vi "GetGraphics.vi"(0 "LcPictureBox in":refnum<class "LcPictureBox.lvclass">, 5 "error in (no error)":errorcluster, 8 "SmoothingMode":T1) -> (14 "LcPictureBox out":refnum<class "LcPictureBox.lvclass">, 16 "Graphics":refnum<k24>, 17 "Scale":dbl, 18 "Offset":cluster{"x":sgl, "y":sgl}, 19 "error out":errorcluster)   [LabVIEW 2020, in "LcPictureBox.lvclass"]
uses:
  LcPictureBox.lvclass
  System.Drawing
  SmoothingMode.ctl
  LcPictureBox.lvclass/LcPictureBox.ctl
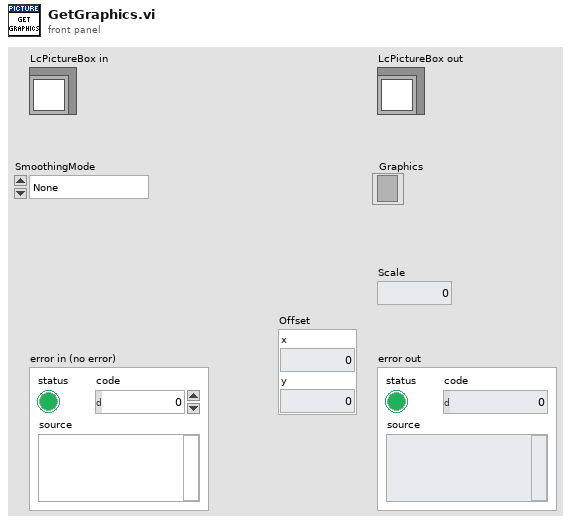
[diagram p1: front panel]
types:
  T1 = typedef "LcPictureBox.lvclass/SmoothingMode.ctl" = enum16{"None", "HighSpeed", "HighQuality", "AntiAlias"}
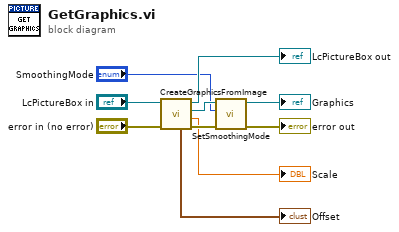
[diagram p0: block diagram]
diagram:
  n1 = call "CreateGraphicsFromImage.vi"("error in (no error)"="error in (no error)", "LcPictureBox in"="LcPictureBox in") -> ("error out"=w8:errorcluster, "Scale"=→"Scale":dbl, "Graphics"=w10:refnum<k24>, "LcPictureBox out"=→"LcPictureBox out":refnum<class "LcPictureBox.lvclass">, "Offset"=→"Offset":cluster{"x":sgl, "y":sgl})  [unwired: 5 in]
  n2 = call "SetSmoothingMode.vi"("error in (no error)"=w8, "SmoothingMode"="SmoothingMode", "CreateGraphics in"=w10) -> ("error out"=→"error out":errorcluster, "CreateGraphics out"=→"Graphics":refnum<k24>)  [unwired: 7 in]
